vi "Invoke Measure Logic.vi"(1 "gRPC ID in":T4, 5 "measurement plugin service in":refnum<class "Measurement Plugin Service.lvclass">, 7 "measurement service in":refnum<class "IMeasurement Service.lvclass">, 9 "measure request":T1, 11 "error in":errorcluster) -> (6 "measure response":T5, 15 "error out":errorcluster)   [LabVIEW 2020, in "Measurement Plugin Measurement Server.lvlib" / "IMeasurement Service.lvclass"]
uses:
  IMeasurement Service.lvclass
  Helpers/TypeDefs/Measure Response.ctl
  Measurement Plugin Measurement Server Internal/RPC Messages/google_protobuf_Any.ctl
  Measurement Plugin Service/Measurement Plugin Service.lvclass
  <vilib>/gRPC/LabVIEW gRPC Library/Shared/grpcId.ctl
  Helpers/TypeDefs/Measure Request.ctl
  <vilib>/gRPC/LabVIEW gRPC Library/Shared/Any.ctl
  Helpers/TypeDefs/Pin Map Context.ctl
  <vilib>/gRPC/LabVIEW gRPC Library/Server API/typeDefs/gRPC Status Code.ctl
  <vilib>/Utility/error.llb/DialogType.ctl
  Measure Call Context/Measure Call Context.lvclass
  <vilib>/gRPC/LabVIEW gRPC Library/grpc-lvsupport-release.lvlib
  Measurement Plugin Measurement Server Internal/Measurement Plugin Measurement Server Internal.lvlib
  Measurement Plugin Measurement Server.lvlib
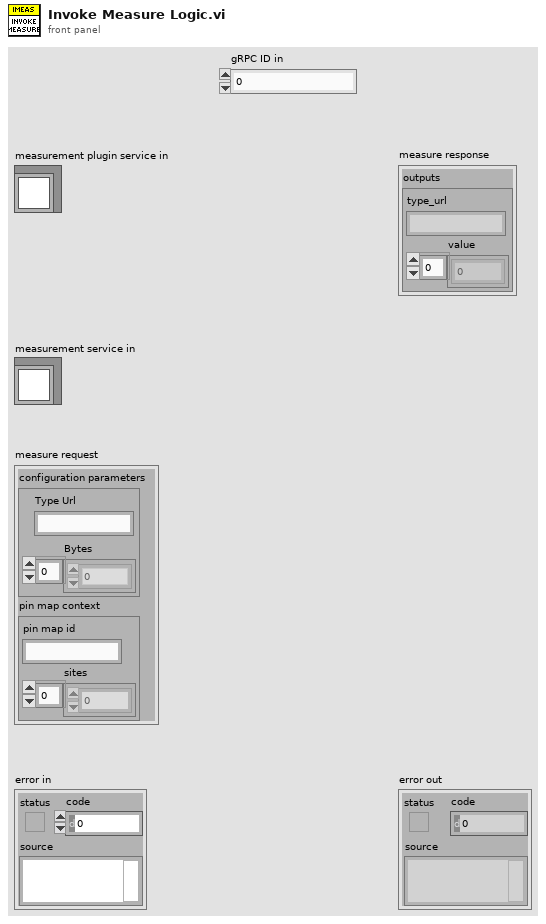
[diagram p1: front panel]
types:
  T1 = typedef "Measurement Plugin Measurement Server.lvlib/Measure Request.ctl" = cluster{"configuration parameters":T2, "pin map context":T3}
  T2 = typedef "grpc-lvsupport-release.lvlib/Any.ctl" = cluster{"Type Url":string, "Bytes":u8[]}
  T3 = typedef "Measurement Plugin Measurement Server.lvlib/Pin Map Context.ctl" = cluster{"pin map id":string, "sites":i32[]}
  T4 = typedef "grpc-lvsupport-release.lvlib/grpcId.ctl" = u64
  T5 = typedef "Measurement Plugin Measurement Server.lvlib/Measure Response.ctl" = cluster{"outputs":T6}
  T6 = typedef "Measurement Plugin Measurement Server Internal.lvlib/google_protobuf_Any.ctl" = cluster{"type_url":string, "value":u8[]}
  T7 = typedef "grpc-lvsupport-release.lvlib/gRPC Status Code.ctl" = enum16{"OK", "CANCELLED", "UNKNOWN", "INVALID_ARGUMENT", "DEADLINE_EXCEEDED", "NOT_FOUND", "ALREADY_EXISTS", "PERMISSION_DENIED", "RESOURCE_EXHAUSTED", "FAILED_PRECONDITION", "ABORTED", "OUT_OF_RANGE", "UNIMPLEMENTED", "INTERNAL", "UNAVAILABLE", "DATA_LOSS", "UNAUTHENTICATED"}
  T8 = typedef "Measurement Plugin Measurement Server.lvlib/Measurement Plugin Service.lvclass/Plugin Paths.ctl" = cluster{"get measurement details VI path":path, "get type specializations VI path":path, "get UI details VI path":path, "measurement logic VI path":path, "measurement configuration ctl path":path, "measurement results ctl path":path}
  T9 = typedef "DialogType.ctl" = u16
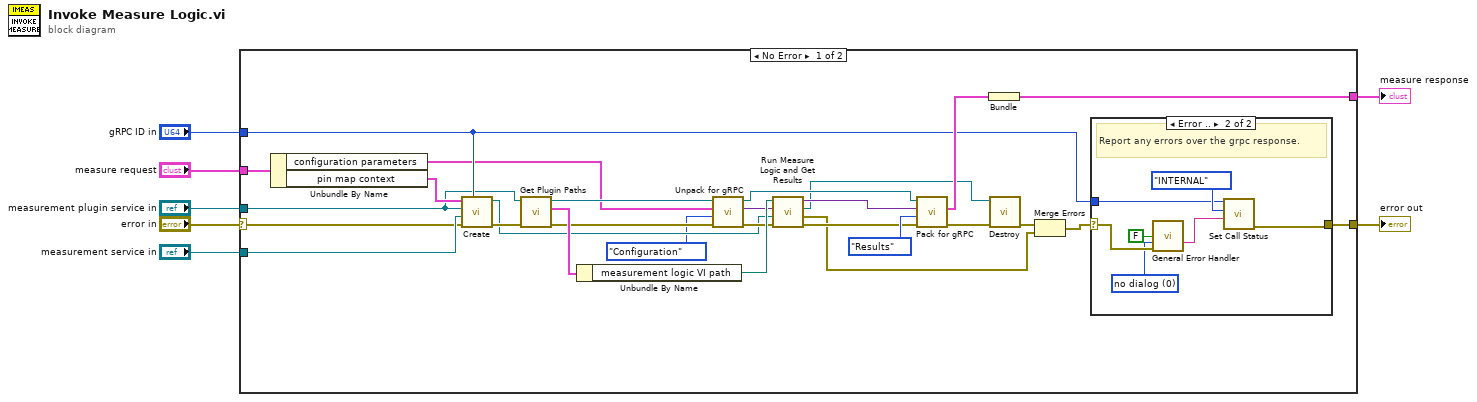
[diagram p0: block diagram]
diagram:
  n1 = case shown="No Error" "error in" {
    selector: "error in" -> [w21 w44]
    tunnel: [w28 w44] -> w6
    tunnel: [w30 _] -> w5
    tunnel: "gRPC ID in" -> [w27 _]
    tunnel: "measurement plugin service in" -> [w12 _]
    tunnel: "measure request" -> [w29 _]
    tunnel: "measurement service in" -> [w26 _]
    frame No Error {
      n2 = Unbundle By Name(w29) -> ("configuration parameters"=w14:T2, "pin map context"=w35:T3)
      n3 = call "Create.vi"("gRPC server ID"=w27, "error in"=w21, "measurement service in"=w26, "measurement plugin service in"=w12, "pin map context"=w35) -> ("error out"=w34:errorcluster, "measure call context out"=w18:refnum<class "Measure Call Context.lvclass">)  [unwired: 5 in]
      n4 = call-dynamic "Get Plugin Paths.vi"("error in"=w34, "measurement plugin service in"=w12) -> ("error out"=w20:errorcluster, "plugin paths"=w31:T8, "measurement plugin service out"=w16:refnum<class "Measurement Plugin Service.lvclass">)  [unwired: 7 in]
      n5 = Unbundle By Name(w31) -> ("measurement logic VI path"=w24:path)
      n6 = call-dynamic "Unpack for gRPC.vi"("error in"=w20, "configuration / results"=enum16{"Configuration", "Results"}."Configuration" ("Configuration / Resuls (Config)"), "any"=w14, "measurement plugin service in"=w16) -> ("error out"=w19:errorcluster, "data value"=w17:variant, "measurement plugin service out"=w15:refnum<class "Measurement Plugin Service.lvclass">)  [unwired: 5 in]
      n7 = call "Run Measure Logic and Get Results.vi"("error in"=w19, "measure call context in"=w18, "measurement configuration"=w17, "measurement logic vi path"=w24) -> ("error out"=w23:errorcluster, "measurement error"=w8:errorcluster, "measure call context out"=w10:refnum<class "Measure Call Context.lvclass">, "measurement output"=w11:variant)  [unwired: 4 in]
      n8 = call-dynamic "Pack for gRPC.vi"("error in"=w23, "configuration / results"=enum16{"Configuration", "Results"}."Results" ("Configuration / Resuls (Config)"), "data value"=w11, "measurement plugin service in"=w15) -> ("error out"=w25:errorcluster, "any"=w33:T2)  [unwired: 5 in, 1 out]
      n9 = Bundle("any"=w33) -> (w30:cluster{"any":T2})  [unwired: 1 in]
      n10 = call "Destroy.vi"("error in"=w25, "measurement context in"=w10) -> ("error out"=w22:errorcluster)  [unwired: 9 in]
      n11 = Merge Errors(w22, w8) -> (w9:errorcluster)
      n12 = case shown="Error .." w9 {
        selector: w9 -> [w36 w40]
        tunnel: [w36 w42] -> w28
        tunnel: w27 -> [_ w41]
        frame No Error {
          # "no error: pass through"
        }
        frame Error {
          w38 = T9 0 items=["no dialog", "OK message", "continue or stop message", "OK message + warnings", "continue/stop + warnings"] ("type of dialog (OK msg:1)")
          # "Report any errors over the grpc response."
          n13 = call <vilib>:"General Error Handler.vi"("search ni.com link visible?(T)"=FALSE, "type of dialog (OK msg:1)"=w38, "error in (no error)"=w40) -> ("message"=w39:string)  [unwired: 8 in, 4 out]
          n14 = call <vilib>:"Set Call Status.vi"("Details"=w39, "Status Code"=gRPC_Status_Code."INTERNAL", "gRPCid in"=w41) -> ("error out"=w42:errorcluster)  [unwired: 7 in, 1 out]
        }
      }
    }
    frame Error {
    }
  }
  "error out" <- w6
  "measure response" <- w5
